vi "Periodic Tasks.vi"(8 "error in":errorcluster) -> ()   [LabVIEW 2015]
doc: "This VI runs in parallel to other tasks. It can contain as many user-defined periodic loops as you need. These can carry out PID or other sorts of timed response."
uses:
  Library/REV Digit MXP/LabVIEW/Brightness.ctl
  Library/REV Digit MXP/LabVIEW/Blink Rate.ctl
  Library/REV Digit MXP/LabVIEW/Display.ctl
  Library/REV Digit MXP/LabVIEW/Oscillator.ctl
panel:
  out "B Pressed":bool
  out "A Pressed":bool
  out "Value (0-1)":dbl
  in  "Diplay":T1
  in  "Blink":T2
  in  "Set Brightness":T3
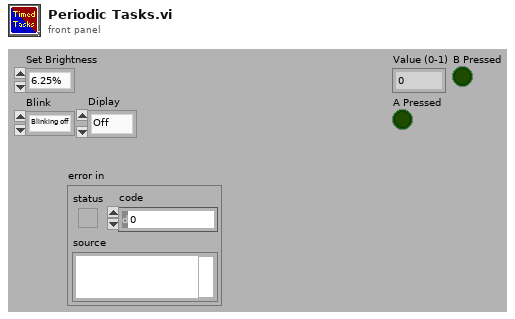
[diagram p1: front panel]
types:
  T1 = typedef "Display.ctl" = enum16{"Off", "On"}
  T2 = typedef "Blink Rate.ctl" = enum16{"Blinking off", "2 Hz", "1 Hz", "0.5 Hz"}
  T3 = typedef "Brightness.ctl" = enum16{"6.25%", "12.5%", "18.75%", "25%", "31.25%", "37.5%", "43.74%", "50%", "56.25%", "62.5%", "68.75%", "75%", "81.25%", "87.5%", "93.75%", "100%"}
  T4 = typedef "Oscillator.ctl" = enum16{"Off", "On"}
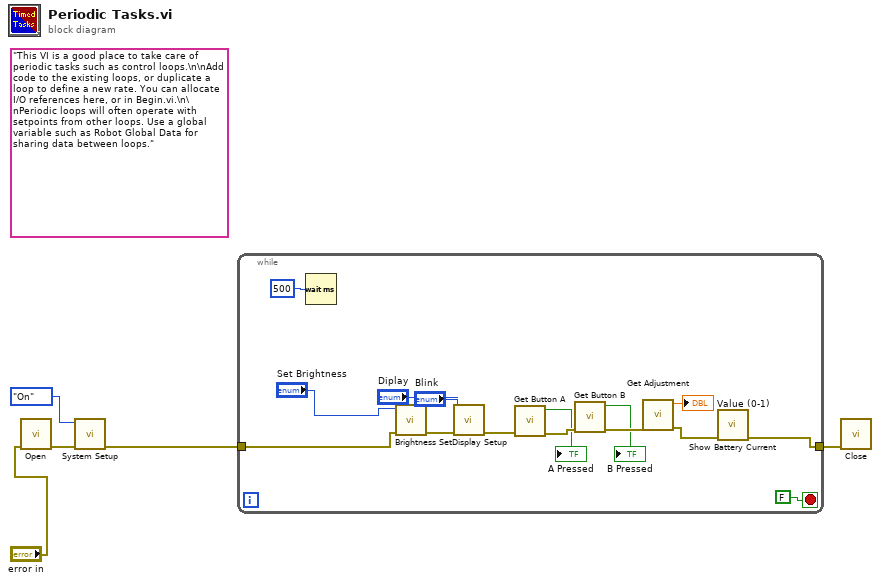
[diagram p0: block diagram]
diagram:
  (unwired) "This VI is a good place to take care of periodic tasks such as control loops.\n\nAdd code to the existing loops, or duplicate a loop to define a new rate. You can allocate I/O references here, or in Begin.vi.\n\nPeriodic loops will often operate with setpoints from other loops. Use a global variable such as Robot Global Data for sharing data between loops."
  n1 = call "Open.vi"("error in (no error)"="error in") -> ("error out"=w4:errorcluster)  [unwired: 10 in]
  n2 = call "System Setup.vi"("error in (no error)"=w4, "Set Oscillator"=Oscillator."On") -> ("error out"=w2:errorcluster)  [unwired: 9 in]
  n3 = while {
    tunnel: [w18] -> w3
    tunnel: w2 -> [w16]
    stop <- FALSE stop-if-true
    n4 = Wait (ms)(milliseconds to wait=u32 500) -> ()  [unwired: 1 out]
    n5 = call "Brightness Set.vi"("error in (no error)"=w16, "Set Brightness"="Set Brightness") -> ("error out"=w17:errorcluster)  [unwired: 9 in]
    n6 = call "Display Setup.vi"("error in (no error)"=w17, "Diplay"="Diplay", "Blink"="Blink") -> ("error out"=w12:errorcluster)  [unwired: 8 in]
    n7 = call "Get Button A.vi"("error in (no error)"=w12) -> ("error out"=w11:errorcluster, "A Pressed"=→"A Pressed":bool)  [unwired: 9 in]
    n8 = call "Get Button B.vi"("error in (no error)"=w11) -> ("error out"=w10:errorcluster, "B Pressed"=→"B Pressed":bool)  [unwired: 9 in]
    n9 = call "Get Adjustment.vi"("error in (no error)"=w10) -> ("error out"=w9:errorcluster, "Adjustment Value (0-1)"=→"Value (0-1)":dbl)  [unwired: 9 in]
    n10 = call "Show Battery Current.vi"("error in (no error)"=w9) -> ("error out"=w18:errorcluster)  [unwired: 10 in]
  }
  n11 = call "Close.vi"("error in (no error)"=w3) -> ()  [unwired: 10 in, 1 out]
